vi "SaveStepToFile.vi"(10 "base path":path, 11 "Step":T1) -> ()   [LabVIEW 2015]
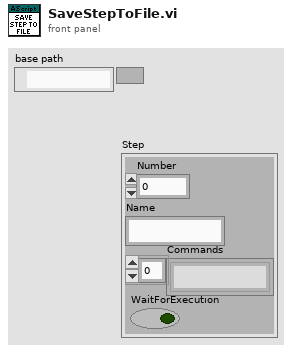
[diagram p1: front panel]
types:
  T1 = cluster{"Number":i32, "Name":string, "Commands":string[], "WaitForExecution":bool}
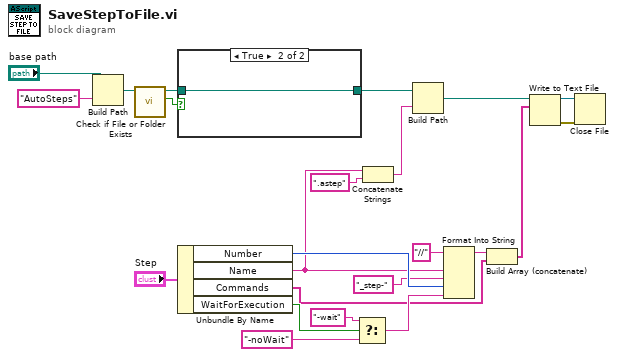
[diagram p0: block diagram]
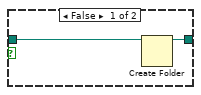
[diagram p2: hidden frame]
diagram:
  n1 = Build Path(base path="base path", name or relative path="AutoSteps") -> (appended path=w20:path)
  n2 = call <vilib>:"Check if File or Folder Exists.vi"("path"=w20) -> ("file or folder exists?"=w23:bool, "dup path"=w22:path)  [unwired: 8 in, 1 out]
  n3 = case shown="True" w23 {
    tunnel: w22 -> [w25 w26]
    tunnel: [w24 w26] -> w6
    frame False {
      n4 = Create Folder(path (use dialog)=w25) -> (created path=w24:path)  [unwired: 2 in, 2 out]
    }
    frame True {
    }
  }
  n5 = Unbundle By Name("Step") -> ("Number"=w14:i32, "Name"=w11:string, "Commands"=w8:string[], "WaitForExecution"=w18:bool)
  n6 = Select(t="-wait", s=w18, f="-noWait") -> (s? t:f=w16:string)
  n7 = Concatenate Strings(w11, ".astep" ("string")) -> (w7:string)
  n8 = Build Path(base path=w6, name or relative path=w7) -> (appended path=w4:path)
  n9 = Format Into String(initial string="//", w11, "_step-" ("input 2"), w14, w16) -> (resulting string=w9:string)  [unwired: 2 in, 1 out]
  n10 = Build Array (concatenate)(w9, w8) -> (w5:string[])
  n11 = Write to Text File(file (use dialog)=w4, text=w5) -> (refnum out=w2:refnum<file>, error out=w3:errorcluster)  [unwired: 2 in, 1 out]
  n12 = Close File(refnum=w2, error in=w3) -> ()  [unwired: 2 out]
